vi "DrawCutImg-LumColorTest.vi"(1 "PosArray":cluster{"P_X":i32, "P_Y":i32}[][](array[cluster]), 2 "Image Out 2":T1, 3 "DrawCut Img":bool) -> (0 "Image Out":T1)   [LabVIEW 2014]
uses:
  <vilib>/vision/Image Controls.llb/IMAQ Image.ctl
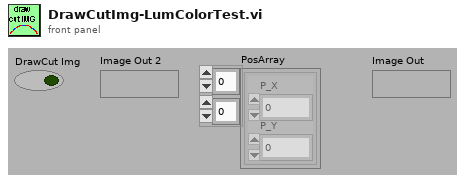
[diagram p1: front panel]
types:
  T1 = typedef "IMAQ Image.ctl" = refnum<image>
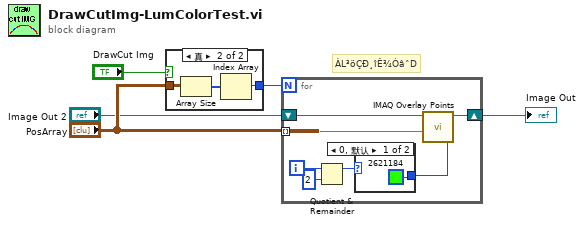
[diagram p0: block diagram]
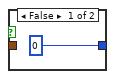
[diagram p2: hidden frame]
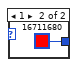
[diagram p3: hidden frame]
diagram:
  # "ÀL³öÇÐ¸îÊ¾ÒâˆD"
  n1 = case shown="真" "DrawCut Img" {
    tunnel: "PosArray" -> [_ w9]
    tunnel: [0 w7] -> w4
    frame False {
    }
    frame True {
      n2 = Array Size(array=w9) -> (size(s)=w8:i32[])
      n3 = Index Array(array=w8) -> (element=w7:i32)  [unwired: 1 in]
    }
  }
  n4 = for {
    N: w4 -> [_]
    shift-right: [w15] -> w2
    shift-left: "Image Out 2" -> [w16]
    tunnel: "PosArray" -> [w10] mode=indexing
    i -> [w13]
    n5 = Quotient & Remainder(x=w13, y=2) -> (x-y*floor(x/y)=w11:i32)  [unwired: 1 out]
    n6 = case shown="0, 默认" w11 {
      tunnel: [u32 2621184 ("Color") u32 16711680 ("Color")] -> w14
      frame 0, Default {
      }
      frame 1 {
      }
    }
    n7 = call "IMAQ Overlay Points"("Color"=w14, "Array of Points"=w10, "Image"=w16) -> ("Image Out"=w15:T1)  [unwired: 3 in, 5 out]
  }
  "Image Out" <- w2
